vi "MainFullCode.vi"() -> ()   [LabVIEW 2018]
uses:
  <vilib>/rvi/interface/nirviOpenFPGA/nirviOpenFPGA.xnode
  <vilib>/rvi/interface/nirviMethod/nirviMethod.xnode
  <vilib>/FPGAPlugInAG/Dynamic/niLvFpga_Run_Dynamic.vi
  <vilib>/Utility/error.llb/DialogType.ctl
  <vilib>/rvi/interface/nirviCloseFPGA/nirviCloseFPGA.xnode
  <vilib>/FPGAPlugInAG/Dynamic/niLvFpga_Close_Dynamic.vi
  <vilib>/FPGAPlugInAG/Dynamic/niLvFpga_Abort_Dynamic.vi
  FPGA Bitfiles/2019HyperXiteCom_FPGATarget_Fail-SafeControl_eg2p2q-h5Jg.lvbitx
  <vilib>/FPGAPlugInAG/cRIO-9063/niLvFpga_Open_cRIO-9063.vi
  <vilib>/rvi/interface/common/dynamic/niFpgaDynamicAddResources.vi
panel:
  out "error out":errorcluster
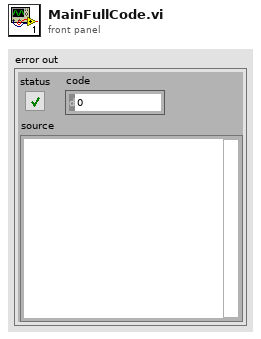
[diagram p1: front panel]
types:
  T1 = typedef "DialogType.ctl" = u16
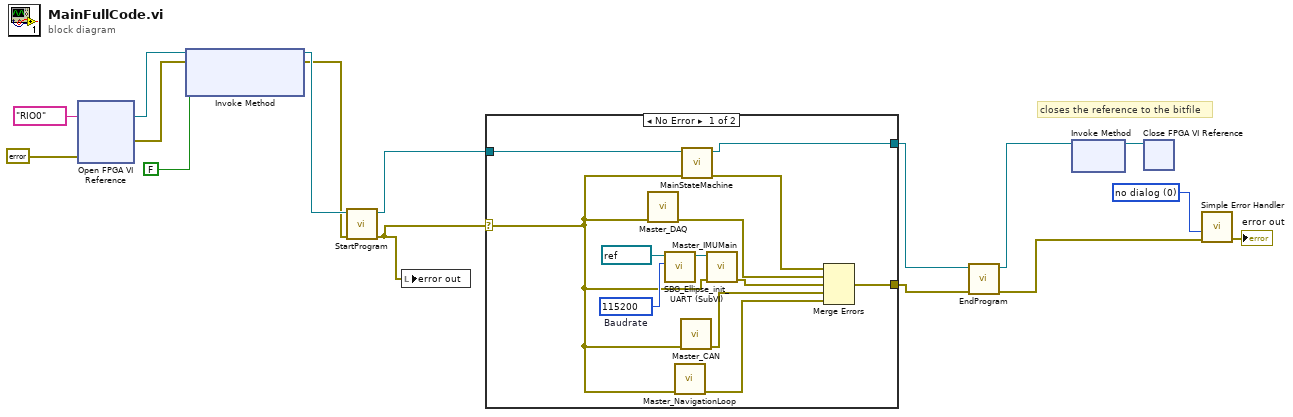
[diagram p0: block diagram]
diagram:
  w8 = T1 0 items=["no dialog", "OK message", "continue or stop message", "OK message + warnings", "continue/stop + warnings"] ("type of dialog (OK msg:1)")
  # "closes the reference to the bitfile"
  n1 = xnode "Open FPGA VI Reference"("error in"=errorcluster {"status"=FALSE, "code"=0, "source"=""}, "resource name"=tag "RIO0") -> ("FPGA VI Reference Out"=w12:refnum<k20>, "error out"=w14:errorcluster)
  n2 = xnode "Invoke Method"("FPGA VI Reference In"=w12, "error in"=w14, "Wait Until Done (F)"=FALSE) -> ("FPGA VI Reference Out"=w10:refnum<k20>, "error out"=w9:errorcluster)
  n3 = call "StartProgram.vi"("error in (no error)"=w9, "FPGA VI Reference In"=w10) -> ("error out"=w5:errorcluster, "FPGA VI Reference out"=w16:refnum<k20>)  [unwired: 8 in]
  n4 = local write "error out"(w5) -> ()
  n5 = case shown="No Error" w5 {
    selector: w5 -> [w19 w30]
    tunnel: [w20 w30] -> w2
    tunnel: w16 -> [w18 w29]
    tunnel: [w17 w29] -> w4
    frame No Error {
      w27 = u32 115200 items=["9600"=9600, "19200"=19200, "36400"=36400, "57600"=57600, "115200"=115200, "230400"=230400, "460800"=460800, "921600"=921600]  # Baudrate
      n6 = call "Master_DAQ.vi"("error in (no error)"=w19) -> ("error out"=w24:errorcluster)  [unwired: 10 in]
      n7 = call "SBG_Ellipse_init_UART (SubVI).vi"("Baudrate"=w27, "VISA Refnum in"=refnum<visa-resource-name> "IMU" ("VISA resource name")) -> ("VISA Refnum out"=w28:refnum<visa-resource-name>)  [unwired: 8 in, 1 out]
      n8 = call "Master_NavigationLoop.vi"("error in (no error)"=w19) -> ("error out"=w21:errorcluster)  [unwired: 10 in]
      n9 = call "Master_CAN.vi"("error in"=w19) -> ("error out"=w22:errorcluster)  [unwired: 10 in]
      n10 = call "MainStateMachine.vi"("error constant"=w19, "FPGA VI Reference In"=w18) -> ("error constant 2"=w25:errorcluster, "FPGA VI Reference Out"=w17:refnum<k20>)  [unwired: 8 in]
      n11 = call "Master_IMUMain.vi"("error in"=w19, "VISA Refnum out"=w28) -> ("error out"=w23:errorcluster)  [unwired: 9 in]
      n12 = Merge Errors(w25, w24, w23, w22, w21) -> (w20:errorcluster)
    }
    frame Error {
    }
  }
  n13 = call "EndProgram.vi"("error in"=w2, "FPGA VI Reference In"=w4) -> ("error out"=w1:errorcluster, "FPGA VI Reference Out"=w3:refnum<k20>)  [unwired: 8 in]
  n14 = xnode "Invoke Method"("FPGA VI Reference In"=w3) -> ("FPGA VI Reference Out"=w7:refnum<k20>)  [unwired: 1 in, 1 out]
  n15 = xnode "Close FPGA VI Reference"("FPGA VI Reference In"=w7) -> ()  [unwired: 1 in, 1 out]
  n16 = call <vilib>:"Simple Error Handler.vi"("type of dialog (OK msg:1)"=w8, "error in (no error)"=w1) -> ("error out"=→"error out":errorcluster)  [unwired: 3 in, 4 out]
